vi "Teleop.vi"(10 "Match Info":T1={"Autonomous Elapsed Seconds"=0.0, "TeleOp Elapsed Seconds"=0.0, "Disabled Elapsed Seconds"=0.0, "Visited Autonomous"=FALSE, "Visited TeleOp"=FALSE, "Visited Disabled"=FALSE, "Autonomous Settings"={"Autonomous Style"=enum."Independent", "VI Refnum"=refnum}}, 11 "Call Context":T2) -> ()   [LabVIEW 2020]
doc: "This VI is called for each TeleOp packet received from the DS where the robot is not disabled. It is often used to read from the joysticks and update I/O or to update setpoints for timed control loops. It should complete and return within 20 milliseconds or it may miss DS packets."
uses:
  <vilib>/Rock Robotics/Network Tables/NT Read Boolean.vi
  <vilib>/Rock Robotics/WPI/ThirdParty/Phoenix-LabVIEW/Motor Controller/Controls/CTRE_Phoenix_MotorControl_ControlMode.ctl
  <vilib>/Rock Robotics/Network Tables/NT Write Boolean.vi
  <vilib>/Rock Robotics/Network Tables/NT Read Number.vi
  TitanLib/Lib/TitanLib.lvlib
  TitanLib/Lib/Piston Hold.vi
  <vilib>/Rock Robotics/WPI/Solenoid/WPI_SolenoidSetEnum.vi
  <vilib>/Rock Robotics/WPI/DriverStation/WPI_DriverStationMatch Info.ctl
  <vilib>/Rock Robotics/WPI/DriverStation/WPI_DriverStationDerivedRobotMode.ctl
panel:
  out "Filtered Waveform Chart":i16(graph)
  out "FIltered SIgnal":i16[](array[numeric])
  out "IR Waveform Output 2":i16[](array[numeric])
  out "Waveform Chart":i16(graph)
  out "Sample Slider 0":dbl(slide) scale=0.0..5.0
  out "Sample Boolean 1":bool
  out "Sample Boolean 0":bool
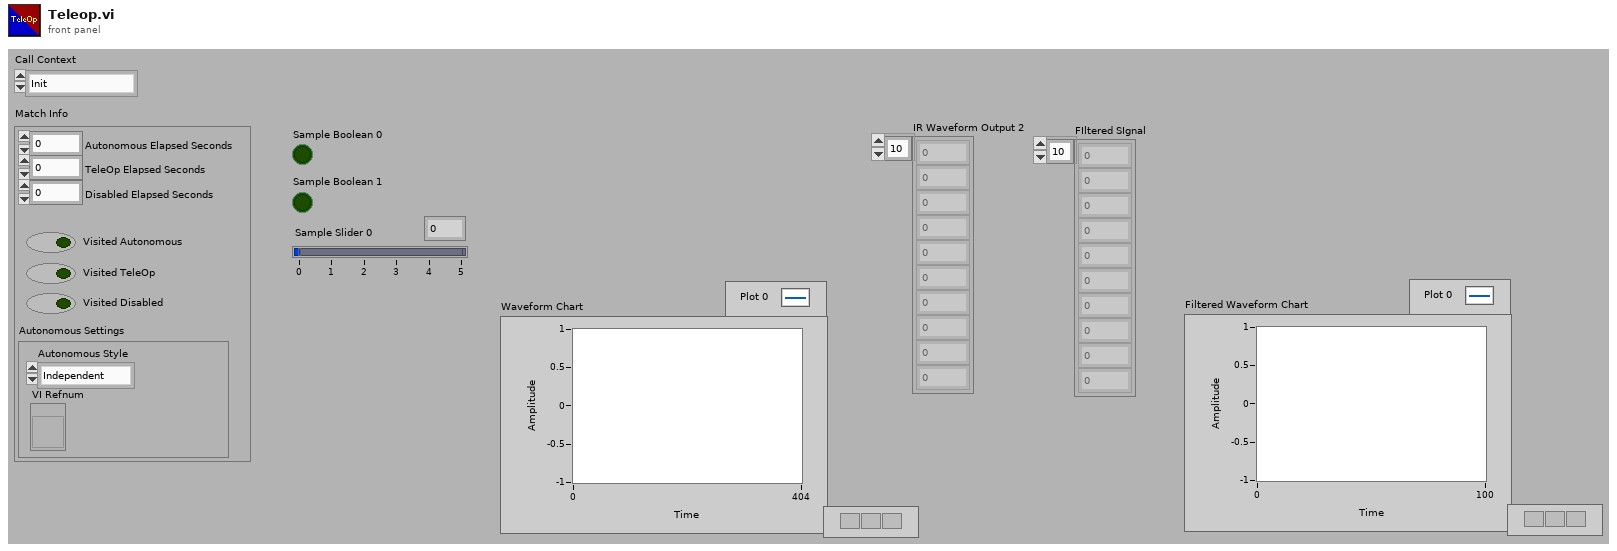
[diagram p1: front panel]
types:
  T1 = typedef "WPI_DriverStationMatch Info.ctl" = cluster{"Autonomous Elapsed Seconds":dbl, "TeleOp Elapsed Seconds":dbl, "Disabled Elapsed Seconds":dbl, "Visited Autonomous":bool, "Visited TeleOp":bool, "Visited Disabled":bool, "Autonomous Settings":cluster{"Autonomous Style":enum16{"Iterative", "Independent"}, "VI Refnum":refnum<vi>}}
  T2 = typedef "WPI_DriverStationDerivedRobotMode.ctl" = enum16{"Init", "Execute", "Stop"}
  T3 = typedef "CTRE_Phoenix_MotorControl_ControlMode.ctl" = u16
  T4 = typedef "WPI_DigitalInputDevRef.ctl" = cluster{"DevStatus":errorcluster, "DIO Channel":T5}
  T5 = typedef "FPGA_DIOChannel.ctl" = enum8{"DIO 0", "DIO 1", "DIO 2", "DIO 3", "DIO 4", "DIO 5", "DIO 6", "DIO 7", "DIO 8", "DIO 9", "DIO MXP 0", "DIO MXP 1", "DIO MXP 2", "DIO MXP 3", "DIO MXP 4", "DIO MXP 5", "DIO MXP 6", "DIO MXP 7", "DIO MXP 8", "DIO MXP 9", "DIO MXP 10", "DIO MXP 11", "DIO MXP 12", "DIO MXP 13", "DIO MXP 14", "DIO MXP 15", "SPI Port CS1", "SPI Port CS2", "SPI Port CS3", "SPI Port MISO", "SPI Port MOSI", "Invalid"}
  T6 = typedef "WPI_JoystickDevRef.ctl" = cluster{"Device":T7}
  T7 = typedef "WPI_JoystickDeviceEnum.ctl" = enum16{"USB 0", "USB 1", "USB 2", "USB 3", "USB 4", "USB 5"}
  T8 = typedef "WPI_MotorControlDeviceRef.ctl" = cluster{"DeviceStatus":errorcluster, "Type":T9, "PWM":cluster{"PWM Channel":T10, "DeadBand":T11}, "CAN":cluster{"Device Number":u8, "SetOutput VI Ref":variant, "GetOutput VI Ref":variant, "Enable VI Ref":variant, "Disable VI Ref":variant, "Data":variant}, "Invert":bool, "DIO PWM":cluster{"PWM \"Enable\" Channel":T10, "DIOChannel":T5, "PWM Rate":dbl}}
  T9 = typedef "WPI_MotorControlType.ctl" = enum16{"PWM", "CAN", "DIO PWM"}
  T10 = typedef "FPGA_DIOPWMChannel.ctl" = enum8{"PWM 0", "PWM 1", "PWM 2", "PWM 3", "PWM 4", "PWM 5", "PWM 6", "PWM 7", "PWM 8", "PWM 9", "PWM MXP 0", "PWM MXP 1", "PWM MXP 2", "PWM MXP 3", "PWM MXP 4", "PWM MXP 5", "PWM MXP 6", "PWM MXP 7", "PWM MXP 8", "PWM MXP 9", "Invalid"}
  T11 = typedef "WPI_PWMDeadband.ctl" = cluster{"Name":string, "maxPositivePwm":i32, "minPositivePwm":i32, "centerPwm":i32, "maxNegativePwm":i32, "minNegativePwm":i32, "angularRange":u16}
  T12 = typedef "WPI_SolenoidValue.ctl" = enum16{"Off", "On", "Forward", "Reverse"}
  T13 = typedef "WPI_SolenoidDevRef.ctl" = cluster{"DevStatus":errorcluster, "Pneumatics Control Module":u8, "Forward Solenoid Channel":T14, "Reverse Solenoid Channel":T14}
  T14 = typedef "WPI_SolenoidChannel.ctl" = enum8{"Solenoid 0", "Solenoid 1", "Solenoid 2", "Solenoid 3", "Solenoid 4", "Solenoid 5", "Solenoid 6", "Solenoid 7", "Solenoid 8", "Solenoid 9", "Solenoid 10", "Solenoid 11", "Solenoid 12", "Solenoid 13", "Solenoid 14", "Solenoid 15", "Invalid"}
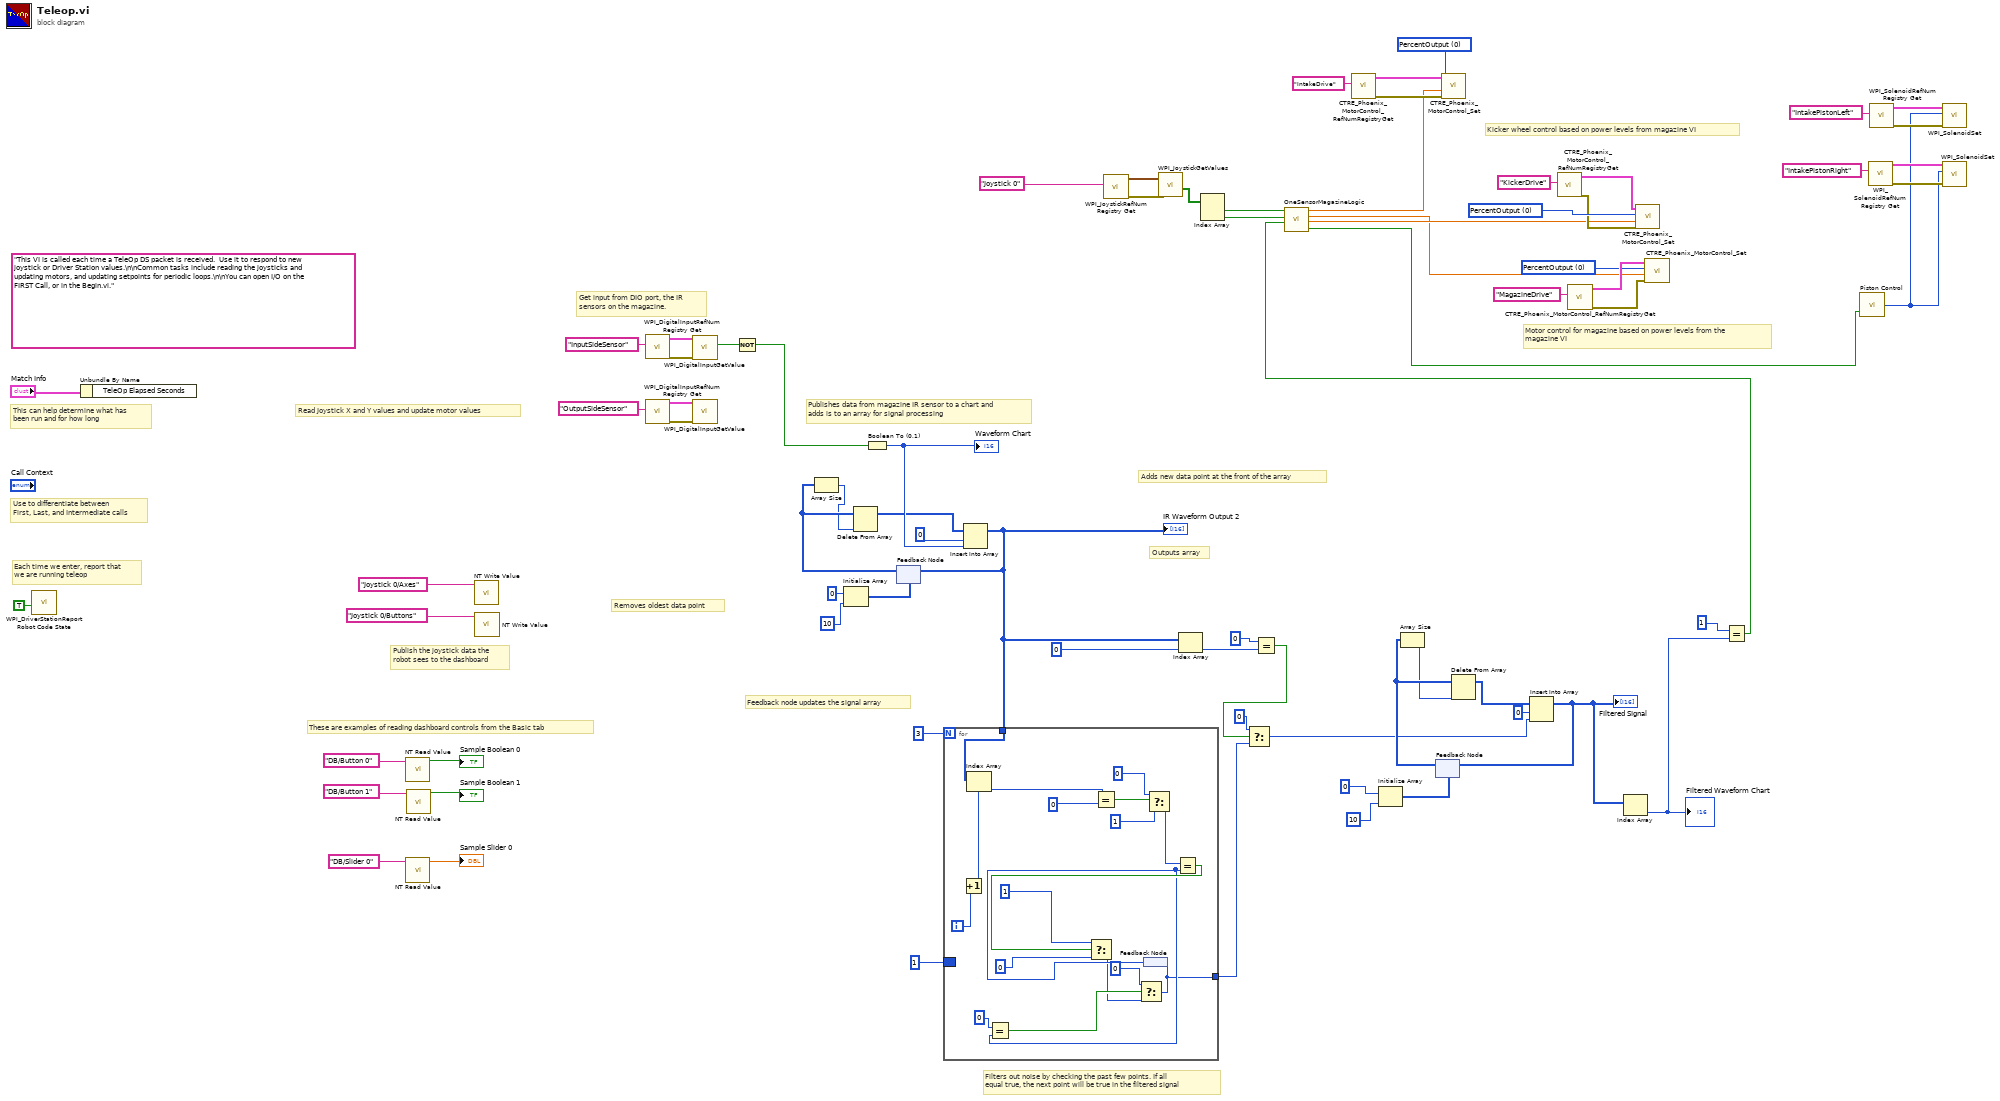
[diagram p0: block diagram]
diagram:
  w16 = T3 0 items=["PercentOutput"=0, "Position"=1, "Velocity"=2, "Current"=3, "Follower"=5, "MotionProfile"=6, "MotionMagic"=7, "MotionProfileArc"=10, "Disabled"=15] ("Control Mode")
  w54 = T3 0 items=["PercentOutput"=0, "Position"=1, "Velocity"=2, "Current"=3, "Follower"=5, "MotionProfile"=6, "MotionMagic"=7, "MotionProfileArc"=10, "Disabled"=15] ("Control Mode")
  w55 = T3 0 items=["PercentOutput"=0, "Position"=1, "Velocity"=2, "Current"=3, "Follower"=5, "MotionProfile"=6, "MotionMagic"=7, "MotionProfileArc"=10, "Disabled"=15] ("Control Mode")
  (unwired) "This VI is called each time a TeleOp DS packet is received.  Use it to respond to new joystick or Driver Station values.\n\nCommon tasks include reading the joysticks and updating motors, and updating setpoints for periodic loops.\n\nYou can open I/O on the FIRST Call, or in the Begin.vi."
  # "Filters out noise by checking the past few points. If all\nequal true, the next point will be true in the filtered signal"
  # "Adds new data point at the front of the array"
  # "Feedback node updates the signal array"
  # "Outputs array"
  # "Removes oldest data point"
  # "Publishes data from magazine IR sensor to a chart and\nadds is to an array for signal processing"
  # "Kicker wheel control based on power levels from magazine VI"
  # "Motor control for magazine based on power levels from the\nmagazine VI"
  # "Get input from DIO port, the IR\nsensors on the magazine."
  # "These are examples of reading dashboard controls from the Basic tab"
  # "Publish the joystick data the\nrobot sees to the dashboard"
  # "Each time we enter, report that\nwe are running teleop"
  # "Use to differentiate between\nFirst, Last, and Intermediate calls"
  # "This can help determine what has\nbeen run and for how long"
  # "Read Joystick X and Y values and update motor values"
  n1 = call <vilib>:"WPI_DriverStationReport Robot Code State.vi"("TeleOp"=TRUE ("Autonomous")) -> ()  [unwired: 10 in, 1 out]
  n2 = Unbundle By Name("Match Info") -> ()  [unwired: 1 out]
  n3 = call-poly <vilib>:"NT Read Value.vi"("Name"="DB/Button 0" ("refnum name")) -> ("Boolean"=→"Sample Boolean 0":bool)  [unwired: 9 in, 1 out]
  n4 = call-poly <vilib>:"NT Read Value.vi"("Name"="DB/Slider 0" ("refnum name")) -> ("Numeric"=→"Sample Slider 0":dbl)  [unwired: 9 in, 1 out]
  n5 = call-poly <vilib>:"NT Read Value.vi"("Name"="DB/Button 1" ("refnum name")) -> ("Boolean"=→"Sample Boolean 1":bool)  [unwired: 9 in, 1 out]
  n6 = call-poly <vilib>:"NT Write Value.vi"("Name"="Joystick 0/Axes") -> ()  [unwired: 10 in, 1 out]
  n7 = call-poly <vilib>:"NT Write Value.vi"("Name"="Joystick 0/Buttons") -> ()  [unwired: 10 in, 1 out]
  n8 = call <vilib>:"WPI_DigitalInputRefNum Registry Get.vi"("refnum name"="InputSideSensor") -> ("error out"=w63:errorcluster, "DigitalInputDevRef"=w62:T4)  [unwired: 9 in]
  n9 = call <vilib>:"WPI_DigitalInputRefNum Registry Get.vi"("refnum name"="OutputSideSensor") -> ("error out"=w61:errorcluster, "DigitalInputDevRef"=w60:T4)  [unwired: 9 in]
  n10 = call <vilib>:"WPI_DigitalInputGetValue.vi"("error in (no error)"=w63, "DigitalInputDevRef"=w62) -> ("Value"=w49:bool)  [unwired: 7 in, 2 out]
  n11 = call <vilib>:"WPI_DigitalInputGetValue.vi"("error in (no error)"=w61, "DigitalInputDevRef"=w60) -> ()  [unwired: 7 in, 3 out]
  n12 = Not(x=w49) -> (.not. x?=w45:bool)
  n13 = Initialize Array(i16 0 ("element"), 10 ("dimension size")) -> (w42:i16[])
  n14 = Boolean To (0,1)(Boolean=w45) -> (0, 1=w48:i16)
  "Waveform Chart" <- w48
  n15 = feedback #1(w42) -> (w41:i16[])
  n16 = Array Size(array=w41) -> (size(s)=w26:i32)
  n17 = Delete From Array(array=w41, index=w26) -> (array with subset deleted=w46:i16[])  [unwired: 1 in, 1 out]
  n18 = Insert Into Array(array=w46, index=0, new element=w48) -> (w27:i16[])
  "IR Waveform Output 2" <- w27
  n19 = feedback-in #1(w27) -> ()
  n20 = for {
    N: 3 -> [_]
    tunnel: w27 -> [w92]
    border: i16 1 ("f") -> [_]
    tunnel: [w77] -> w23
    i -> [w94]
    n21 = Increment(x=w94) -> (x+1=w93:i32)
    n22 = Index Array(array=w92, index=w93) -> (element=w90:i16)
    n23 = Equal?(x=w90, y=i16 0) -> (x = y?=w89:bool)
    n24 = feedback #2() -> (w84:i16)
    n25 = Equal?(x=i16 0, y=w84) -> (x = y?=w82:bool)
    n26 = Select(t=i16 0, s=w89, f=i16 1) -> (s? t:f=w86:i16)
    n27 = Equal?(x=w86, y=w84) -> (x = y?=w85:bool)
    n28 = Select(t=i16 1, s=w85, f=i16 0) -> (s? t:f=w81:i16)
    n29 = Select(t=i16 0, s=w82, f=w81) -> (s? t:f=w77:i16)
    n30 = feedback-in #2(w77) -> ()
  }
  n31 = call <vilib>:"WPI_JoystickRefNum Registry Get.vi"("refnum name"="Joystick 0") -> ("error out"=w65:errorcluster, "JoystickDevRef"=w64:T6)  [unwired: 9 in]
  n32 = call <vilib>:"WPI_JoystickGetValues.vi"("error in (no error)"=w65, "JoystickDevRef"=w64) -> ("Buttons"=w19:bool[])  [unwired: 5 in, 4 out]
  n33 = Index Array(array=w27, index=0) -> (element=w39:i16)
  n34 = Index Array(array=w19) -> (element #1=w14:bool, element #2=w13:bool)  [unwired: 2 in]
  n35 = Equal?(x=i16 0, y=w39) -> (x = y?=w37:bool)
  n36 = Select(t=i16 0, s=w37, f=w23) -> (s? t:f=w29:i16)
  n37 = call <vilib>:"CTRE_Phoenix_MotorControl_RefNumRegistryGet.vi"("refnum name"="IntakeDrive") -> ("error out"=w17:errorcluster, "PhoenixMotorControlDevRef"=w18:T8)  [unwired: 9 in]
  n38 = Initialize Array(i16 0 ("element"), 10 ("dimension size")) -> (w34:i16[])
  n39 = feedback #3(w34) -> (w32:i16[])
  n40 = Array Size(array=w32) -> (size(s)=w25:i32)
  n41 = Delete From Array(array=w32, index=w25) -> (array with subset deleted=w31:i16[])  [unwired: 1 in, 1 out]
  n42 = Insert Into Array(array=w31, index=0, new element=w29) -> (w22:i16[])
  "FIltered SIgnal" <- w22
  n43 = feedback-in #3(w22) -> ()
  n44 = call <vilib>:"CTRE_Phoenix_MotorControl_RefNumRegistryGet.vi"("refnum name"="KickerDrive") -> ("error out"=w52:errorcluster, "PhoenixMotorControlDevRef"=w53:T8)  [unwired: 9 in]
  n45 = call <vilib>:"CTRE_Phoenix_MotorControl_RefNumRegistryGet.vi"("refnum name"="MagazineDrive") -> ("error out"=w56:errorcluster, "PhoenixMotorControlDevRef"=w57:T8)  [unwired: 9 in]
  n46 = Index Array(array=w22) -> (element=w21:i16)  [unwired: 1 in]
  "Filtered Waveform Chart" <- w21
  n47 = Equal?(x=i16 1, y=w21) -> (x = y?=w12:bool)
  n48 = call "OneSensorMagazineLogic.vi"("Intake Side Sensor"=w12, "Outtake Button"=w13, "Intake Toggle"=w14) -> ("Intake Pistons"=w6:bool, "Kicker Motors"=w10:dbl, "Magazine Motors"=w9:dbl, "Intake Motors"=w11:dbl)  [unwired: 1 in]
  n49 = call <vilib>:"CTRE_Phoenix_MotorControl_Set.vi"("error in (no error)"=w17, "Output"=w11, "Control Mode"=w16, "PhoenixMotorControlDevRef"=w18) -> ()  [unwired: 6 in, 2 out]
  n50 = call <vilib>:"CTRE_Phoenix_MotorControl_Set.vi"("error in (no error)"=w52, "Output"=w10, "Control Mode"=w54, "PhoenixMotorControlDevRef"=w53) -> ()  [unwired: 6 in, 2 out]
  n51 = call <vilib>:"CTRE_Phoenix_MotorControl_Set.vi"("error in (no error)"=w56, "Output"=w9, "Control Mode"=w55, "PhoenixMotorControlDevRef"=w57) -> ()  [unwired: 6 in, 2 out]
  n52 = call-poly "Piston Control.vi"("Input"=w6) -> ("Output"=w1:T12)  [unwired: 1 in]
  n53 = call <vilib>:"WPI_SolenoidRefNum Registry Get.vi"("refnum name"="IntakePistonRight") -> ("error out"=w3:errorcluster, "SolenoidDevRef"=w2:T13)  [unwired: 9 in]
  n54 = call <vilib>:"WPI_SolenoidRefNum Registry Get.vi"("refnum name"="IntakePistonLeft") -> ("error out"=w5:errorcluster, "SolenoidDevRef"=w4:T13)  [unwired: 9 in]
  n55 = call-poly <vilib>:"WPI_SolenoidSet.vi"("error in (no error)"=w5, "Value"=w1, "SolenoidDevRef"=w4) -> ()  [unwired: 7 in, 2 out]
  n56 = call-poly <vilib>:"WPI_SolenoidSet.vi"("error in (no error)"=w3, "Value"=w1, "SolenoidDevRef"=w2) -> ()  [unwired: 7 in, 2 out]
